vi "SetRTprotocol.vi"(8 "error in (no error)":errorcluster, 11 "Qbus in":refnum<class "Qbus.lvclass">) -> (0 "error out":errorcluster)   [LabVIEW 2017, in "Controller.lvlib"]
uses:
  <vilib>/addons/InsightCM/Devices/Shared/Common/Controller/Controller.lvlib
  <vilib>/addons/Qbus/Qbus.lvclass
  <vilib>/addons/InsightCM/Utilities/GlobalConfiguration/GlobalConfiguration.lvlib
  <vilib>/addons/InsightCM/Utilities/PropertyHelpers/PropertyHelpers.lvlib
  <vilib>/addons/InsightCM/Utilities/Security/RTProtocol/RTProtocol.lvlib
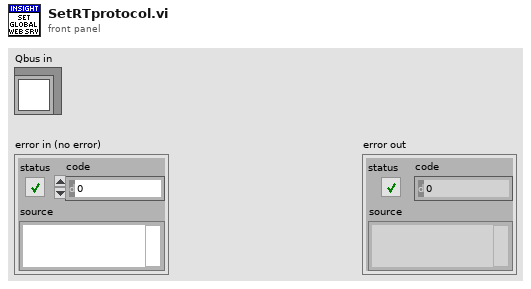
[diagram p1: front panel]
types:
  T1 = typedef "SectionKeyValues.ctl" = cluster{"Section":string, "KeyValues":T2[]}
  T2 = typedef "KeyValuePair.ctl" = cluster{"Key":string, "Value":string}
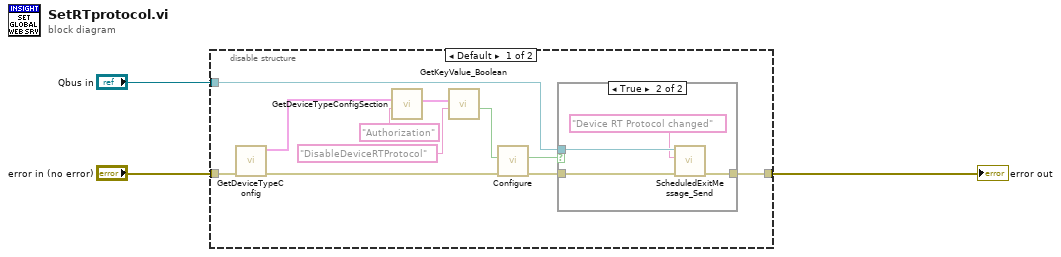
[diagram p0: block diagram]
diagram:
  n1 = disable-structure shown="Default" {
    disable-tunnel: "error in (no error)" -> [w10 w20]
    disable-tunnel: [w5 w20] -> w2
    disable-tunnel: "Qbus in" -> [w4 _]
    frame condition #0 {
      n2 = call <vilib>:"GetDeviceTypeConfig.vi"("error in (no error)"=w10) -> ("error out"=w9:errorcluster, "key values"=w14:T1[])  [unwired: 8 in, 1 out]
      n3 = call <vilib>:"GetDeviceTypeConfigSection.vi"("key"="Authorization", "key values"=w14) -> ("key value pairs out"=w12:T2[])  [unwired: 8 in, 1 out]
      n4 = call <vilib>:"GetKeyValue_Boolean.vi"("key"="DisableDeviceRTProtocol", "key value pairs"=w12) -> ("value"=w8:bool)  [unwired: 7 in, 2 out]
      n5 = call <vilib>:"Configure.vi"("error in (no error)"=w9, "DisableRTProtocol"=w8) -> ("error out"=w6:errorcluster, "reboot required"=w7:bool)  [unwired: 8 in]
      n6 = case shown="True" w7 {
        tunnel: w6 -> [w15 w19]
        tunnel: [w15 w18] -> w5
        tunnel: w4 -> [_ w17]
        frame False {
        }
        frame True {
          n7 = call <vilib>:"ScheduledExitMessage_Send.vi"("error in (no error)"=w19, "scheduled exit reason"="Device RT Protocol changed", "Qbus in"=w17) -> ("error out"=w18:errorcluster)  [unwired: 7 in, 1 out]
        }
      }
    }
    frame condition #1 (active) {
    }
  }
  "error out" <- w2
